vi "Measurement Logic.vi"() -> ()   [LabVIEW 2020, in "Service.lvlib"]
uses:
  Service.lvlib
  Measurement Results.ctl
  <vilib>/Plug-In SDKs/Measurements/Measure Call Context/Measure Call Context.lvclass
  Measurement Configuration.ctl
panel:
  out "measure call context out":refnum<class "Measure Call Context.lvclass">
  in  "measure call context in":refnum<class "Measure Call Context.lvclass">
  out "measurement results":T1
  in  "measurement configuration":T2
  out "error out":errorcluster
  in  "error in":errorcluster
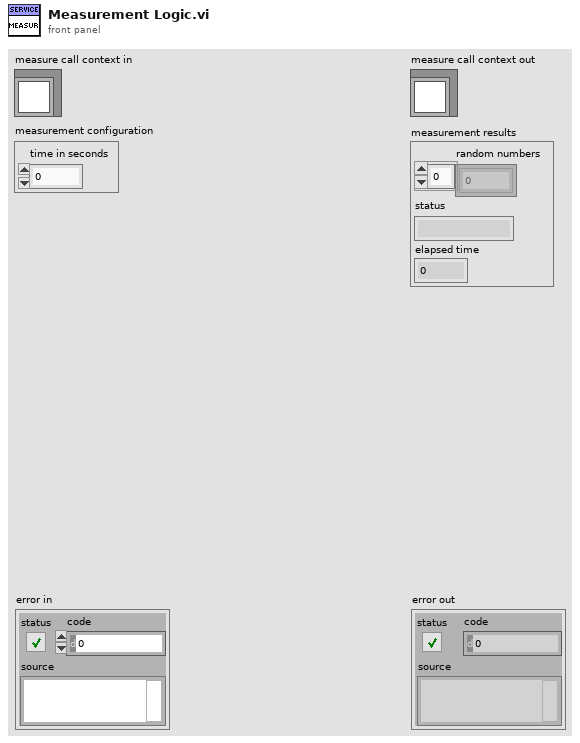
[diagram p1: front panel]
types:
  T1 = typedef "Service.lvlib/Measurement Results.ctl" = cluster{"random numbers":dbl[], "status":string, "elapsed time":dbl}
  T2 = typedef "Service.lvlib/Measurement Configuration.ctl" = cluster{"time in seconds":dbl}
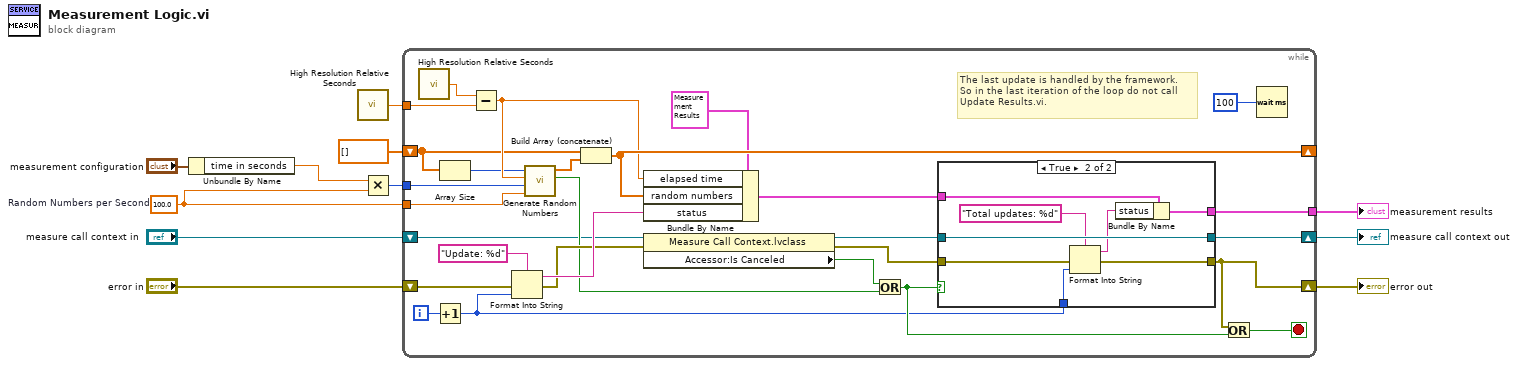
[diagram p0: block diagram]
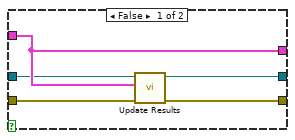
[diagram p2: hidden frame]
diagram:
  w5 = 100.0  # Random Numbers per Second
  n1 = Unbundle By Name("measurement configuration") -> ("time in seconds"=w9:dbl)
  n2 = call <vilib>:"High Resolution Relative Seconds.vi"() -> ("relative seconds"=w8:dbl)
  n3 = Multiply(x=w9, y=w5) -> (x*y=w6:i32)
  n4 = while {
    shift-right: [w33] -> w1
    shift-left: "error in" -> [w39]
    shift-right: [w22] -> _
    shift-left: dbl[] [] -> [w20]
    tunnel: [w29] -> w2
    tunnel: w8 -> [w25]
    tunnel: w5 -> [w16]
    tunnel: w6 -> [w17]
    shift-right: [w13] -> w10
    shift-left: "measure call context in" -> [w15]
    i -> [w28]
    stop <- w30 stop-if-true
    # "The last update is handled by the framework.\nSo in the last iteration of the loop do not call\nUpdate Results.vi."
    n5 = call <vilib>:"High Resolution Relative Seconds.vi"() -> ("relative seconds"=w26:dbl)
    n6 = Increment(x=w28) -> (x+1=w24:i32)
    n7 = Array Size(array=w20) -> (size(s)=w19:i32)
    n8 = Subtract(x=w26, y=w25) -> (x-y=w21:dbl)
    n9 = Format Into String(format string="Update: %d", error in=w39, w24) -> (resulting string=w38:string, error out=w36:errorcluster)  [unwired: 1 in]
    n10 = call "Generate Random Numbers.vi"("random numbers per second"=w16, "stop length"=w17, "elapsed time"=w21, "current array size"=w19) -> ("done?"=w18:bool, "random numbers out"=w31:dbl[])  [unwired: 6 in]
    n11 = Build Array (concatenate)(w20, w31) -> (w22:dbl[])
    n12 = Bundle By Name(cluster=T1 {"random numbers"=[0.012339348035839049, 0.08147256568525073, 0.19559853223976242, 0.2178579491752059, 0.20160852422492445, 0.2052872242185709, 0.3827624603509743, 0.35122322375606946, 0.31347194427565966, 0.38474052913834267, 0.5028374974653135, 0.6135150953796312, 0.5736593207009871, 0.6859575153142563, 0.6583319440852355, 0.6832922138312826, 0.6435805459968538, 0.74420220190326, 0.8534677127358208, 0.7698467429153435, 0.7584629186548848, 0.7955450876816106, 0.7976964250532262, 0.9710855237621672, 1.0166642968878776, 0.9591148837046757, 0.9427124378590327, 1.057050815980074, 0.9169192346904357, 1.0373265903517426, 1.0481481429104984, 0.9644704782136466, 1.0624250558809267, 1.0782966517143304, 1.0655892866080492, 1.0792501716179275, 0.9173606250591974, 1.007297183203816, 0.9231907172397159, 0.9723711254780377, 0.8628784212970436, 0.9565888355525257, 0.9395219608783196, 0.8737093010567047, 0.797390229822592, 0.8489811506284091, 0.8609767867254499, 0.8386861940979295, 0.7891853877158086, 0.6476507318570596, 0.723070530997128, 0.6800546211116898, 0.6131222168201242, 0.6024432443676695, 0.3722593224786126, 0.3857871913902311, 0.322503312034312, 0.39115738119495586, 0.26912575909542613, 0.32352254970681604, 0.22565956921171743, 0.053838470172325, 0.11962900407316593, 0.06710132388297166, 0.07825555037261937, -0.06858407009790907, -0.07419420708872068, -0.22621083209596438, -0.12337183052951747, -0.2563395702834876, -0.2005794491159347, -0.2794921722401782, -0.34597250246868366, -0.5053323132835933, -0.4256354381473161, -0.5473573243588948, -0.49816789862725597, -0.6661751140266309, -0.6670727124701914, -0.5890866112846731, -0.7606879954414798, -0.7157458765605416, -0.7747354812465306, -0.7575048116522464, -0.810896278406414, -0.8460171923361346, -0.9807092523863692, -0.838793478839177, -0.8417627391751608, -1.0145593209993058, -0.9838576974637534, -0.8830147421354331, -0.8962009498018404, -0.9451502309804906, -1.0803966250364196, -0.9493642027781652, -0.9276460732826642, -0.9899412227059524, -1.0397372656478696, -1.027956275705813, -0.9153156403750894, -1.0224755068204006, -0.9685007821133657, -0.9383101845230608, -0.9253207326622068, -0.8201278626442747, -0.9033927618012672, -0.8234139030833569, -0.798472335399, -0.7764491035380428, -0.7258885982132625, -0.7658466116748271, -0.6918185556409187, -0.5862267192894932, -0.6000965489362071, -0.5765845432566191, -0.5368282911308032, -0.43656508168034025, -0.40443271553247945, -0.3747214534723189, -0.2828311353677533, -0.400197442717364, -0.2971397868648525, -0.21222206658595683, -0.15118224029184718, -0.20735730495091192, -0.10741513375653078, 0.0015311036031455671], "status"="", "elapsed time"=0.0} ("Measurement Results"), "elapsed time"=w21, "random numbers"=w22, "status"=w38) -> (w32:T1)
    n13 = property class="Measure Call Context.lvclass"(reference=w15, error in=w36) -> (reference out=w14:refnum<class "Measure Call Context.lvclass">, error out=w35:errorcluster, "Accessor:Is Canceled"=w34:bool)
    n14 = Or(x=w34, y=w18) -> (x .or. y?=w27:bool)
    n15 = case shown="True" w27 {
      tunnel: w14 -> [w40 w52]
      tunnel: w35 -> [w44 w49]
      tunnel: [w41 w52] -> w13
      tunnel: [w43 w48] -> w33
      tunnel: w32 -> [w42 w51]
      tunnel: [w42 w50] -> w29
      tunnel: w24 -> [_ w45]
      frame False {
        n16 = call <vilib>:"Update Results.vi"("error in"=w44, "measurement results"=w42, "measure call context in"=w40) -> ("error out"=w43:errorcluster, "measure call context out"=w41:refnum<class "Measure Call Context.lvclass">)  [unwired: 7 in]
      }
      frame True {
        n17 = Format Into String(format string="Total updates: %d" ("status"), error in=w49, w45) -> (resulting string=w46:string, error out=w48:errorcluster)  [unwired: 1 in]
        n18 = Bundle By Name(cluster=w51, "status"=w46) -> (w50:T1)
      }
    }
    n19 = Or(x=w33, y=w27) -> (x .or. y?=w30:bool)
    n20 = Wait (ms)(milliseconds to wait=u32 100 ("UI Update Interval (msec)")) -> ()  [unwired: 1 out]
  }
  "error out" <- w1
  "measurement results" <- w2
  "measure call context out" <- w10
